vi "Wire Indicators to Mock Call.vi"(8 "error in (no error)":errorcluster, 11 "VI in":refnum<vi>) -> (0 "error out":errorcluster, 3 "VI out":refnum<vi>)   [LabVIEW 2020, in "Responsive Mock Class Generator.lvclass"]
uses:
  Responsive Mock Class Generator.lvclass
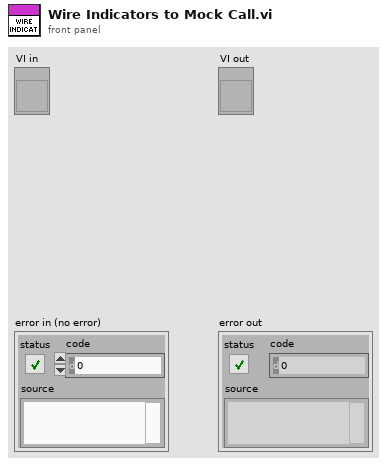
[diagram p1: front panel]
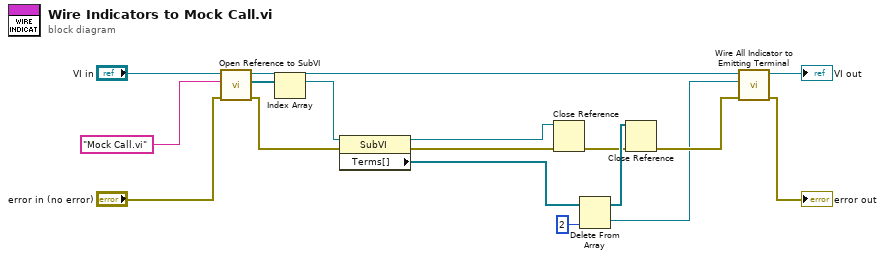
[diagram p0: block diagram]
diagram:
  n1 = call "Open Reference to SubVI.vi"("error in (no error)"="error in (no error)", "SubVI Name"="Mock Call.vi" ("y"), "VI in"="VI in") -> ("error out"=w15:errorcluster, "SubVIs"=w16:refnum<vi>[], "VI out"=w3:refnum<vi>)  [unwired: 6 in]
  n2 = Index Array(array=w16) -> (element=w1:refnum<vi>)  [unwired: 1 in]
  n3 = property class="SubVI"(reference=w1, error in=w15) -> (reference out=w11:refnum<vi>, error out=w10:errorcluster, "Terms[]"=w13:refnum<vi>[])
  n4 = Close Reference(reference=w11, error in (no error)=w10) -> (error out=w9:errorcluster)
  n5 = Delete From Array(array=w13, index=2) -> (deleted portion=w2:refnum<vi>, array with subset deleted=w12:refnum<vi>[])  [unwired: 1 in]
  n6 = Close Reference(reference=w12, error in (no error)=w9) -> (error out=w8:errorcluster)
  n7 = call "Wire All Indicator to Emitting Terminal.vi"("error in (no error)"=w8, "Emitting Terminal"=w2, "VI in"=w3) -> ("error out"=→"error out":errorcluster, "VI out"=→"VI out":refnum<vi>)  [unwired: 7 in]
